vi "filter_detections.vi"(11 "detections":u32[](array[numeric])) -> (3 "filtered":u32[](array[numeric]))   [LabVIEW 2014]
uses:
  <vilib>/Analysis/3filter.llb/FIR Filter (DBL).vi
  <vilib>/Analysis/NI_AALBase.lvlib
panel:
  in  "window_size_ns":i32=100
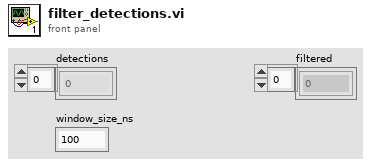
[diagram p1: front panel]
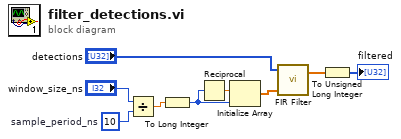
[diagram p0: block diagram]
diagram:
  w5 = 10  # sample_period_ns
  n1 = Divide(x="window_size_ns", y=w5) -> (x/y=w3:dbl)
  n2 = To Long Integer(number=w3) -> (32bit integer=w4:i32)
  n3 = Reciprocal(x=w4) -> (1/x=w8:dbl)
  n4 = Initialize Array(w8, w4) -> (w7:dbl[])
  n5 = call-poly <vilib>:"FIR Filter.vi"("FIR Coefficients"=w7, "X"="detections") -> ("Filtered X"=w9:dbl[])  [unwired: 2 in, 1 out]
  n6 = To Unsigned Long Integer(number=w9) -> (unsigned 32bit integer=→"filtered":u32[])
